vi "getflicker response string.vi"(0 "getflicker response string":string="Flicker : 000.00 %   Flicker index: 0.000000  Flicker frequencies: 000.00 Hz 001.00 Hz\r\n") -> (14 "Flicker %":dbl, 15 "Flicker index":dbl, 16 "Flicker Frequencies 1":dbl, 17 "Flicker Frequencies 2":dbl)   [LabVIEW 2025]
panel:
  out "Flicker Frequencies 2":string
  out "after substring":string
  out "Flicker Frequencies":string
  out "Flicker index":string
  out "Flicker %":string
  # "Flicker : 000.00 %   Flicker index: 0.000000  Flicker frequencies: 000.00 Hz 001.00 Hz"
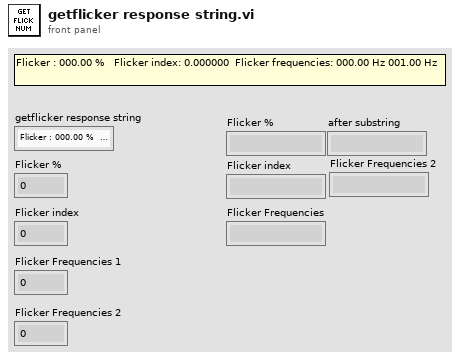
[diagram p1: front panel]
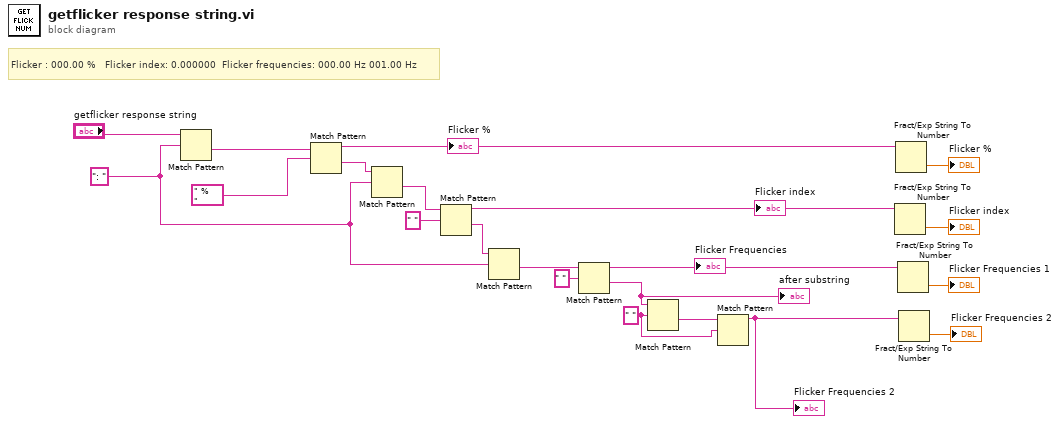
[diagram p0: block diagram]
diagram:
  w9 = " " ("regular expression")
  w15 = ": " ("regular expression")
  # "Flicker : 000.00 %   Flicker index: 0.000000  Flicker frequencies: 000.00 Hz 001.00 Hz"
  n1 = Match Pattern(string="getflicker response string", regular expression=w15) -> (after substring=w17:string)  [unwired: 1 in, 3 out]
  n2 = Match Pattern(string=w17, regular expression=" %   ") -> (before substring=w8:string, after substring=w13:string)  [unwired: 1 in, 2 out]
  "Flicker %" <- w8
  n3 = Match Pattern(string=w13, regular expression=w15) -> (after substring=w16:string)  [unwired: 1 in, 3 out]
  n4 = Match Pattern(string=w16, regular expression=" ") -> (before substring=w7:string, after substring=w12:string)  [unwired: 1 in, 2 out]
  "Flicker index" <- w7
  n5 = Match Pattern(string=w12, regular expression=w15) -> (after substring=w14:string)  [unwired: 1 in, 3 out]
  n6 = Match Pattern(string=w14, regular expression=" ") -> (before substring=w5:string, after substring=w11:string)  [unwired: 1 in, 2 out]
  "Flicker Frequencies" <- w5
  "after substring" <- w11
  n7 = Match Pattern(string=w11, regular expression=w9) -> (after substring=w10:string)  [unwired: 1 in, 3 out]
  n8 = Match Pattern(string=w10, regular expression=w9) -> (before substring=w6:string)  [unwired: 1 in, 3 out]
  "Flicker Frequencies 2" <- w6
  n9 = Fract/Exp String To Number(string=w7) -> (number=→"Flicker index":dbl)  [unwired: 3 in, 1 out]
  n10 = Fract/Exp String To Number(string=w8) -> (number=→"Flicker %":dbl)  [unwired: 3 in, 1 out]
  n11 = Fract/Exp String To Number(string=w5) -> (number=→"Flicker Frequencies 1":dbl)  [unwired: 3 in, 1 out]
  n12 = Fract/Exp String To Number(string=w6) -> (number=→"Flicker Frequencies 2":dbl)  [unwired: 3 in, 1 out]
